vi "CAEN_daisy_isolated.vi"() -> ()   [LabVIEW 2018]
uses:
  <instrlib>/CAEN PSM/CAEN PSM.lvlib
panel:
  in  "Current Limit (0.00 uA)":sgl[](array[numeric]) format="%.2g"
  in  "Voltage Max (0.0 V)":u16[](array[numeric]) max=9999
  in  "Voltage Level (0.0 V)":dbl[](array[numeric]) format="%.1g"
  in  "Apply settings":bool
  out "IMon values (uA)":dbl[](array[numeric])
  out "VMon values (V)":dbl[](array[numeric])
  in  "stop":bool
  in  "VISA resource name":refnum<visa-resource-name>
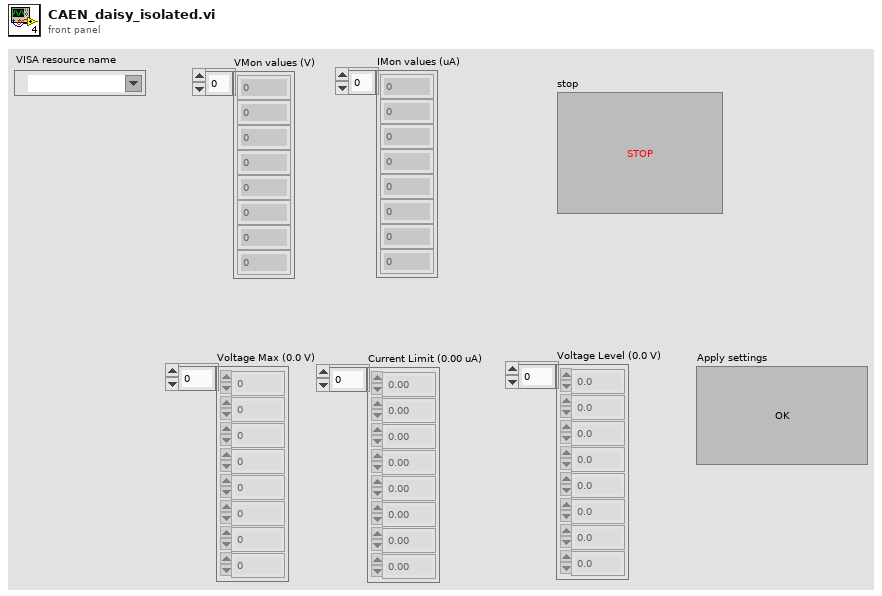
[diagram p1: front panel]
types:
  T1 = typedef "CAEN PSM.lvlib/BoardHandle.ctl" = cluster{"VISA resource name":refnum<visa-resource-name>, "Board address":u8, "NChannels":u8}
  T2 = cluster{"VISA resource name":refnum<visa-resource-name>, "Board address":u8, "NChannels":u8}
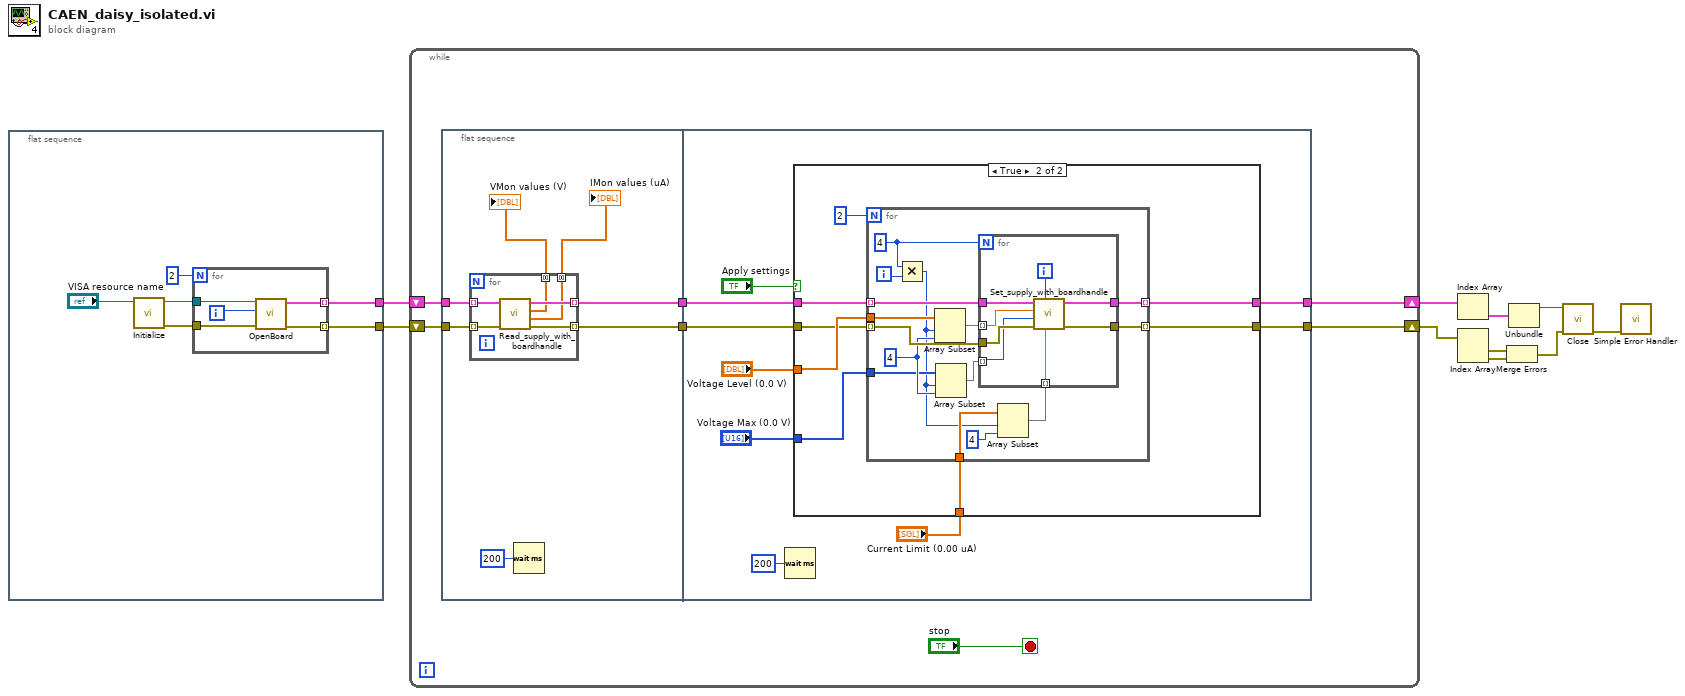
[diagram p0: block diagram]
diagram:
  n1 = flat-sequence {
    tunnel: [w12] -> w10
    tunnel: [w11] -> w9
    frame #0 {
      n2 = call <instrlib>:"Initialize.vi"("VISA resource name"="VISA resource name") -> ("error out"=w14:errorcluster, "VISA resource name out"=w15:refnum<visa-resource-name>)  [unwired: 9 in]
      n3 = for {
        N: 2 -> [_]
        tunnel: w15 -> [w21]
        tunnel: w14 -> [w19]
        tunnel: [w18] -> w11 mode=indexing
        tunnel: [w17] -> w12 mode=indexing
        i -> [w20]
        n4 = call <instrlib>:"OpenBoard.vi"("error in (no error)"=w19, "Board Address"=w20, "VISA resource name"=w21) -> ("error out"=w18:errorcluster, "BoardHandle"=w17:T1)  [unwired: 7 in]
      }
    }
  }
  n5 = while {
    shift-right: [w23] -> w8
    shift-left: w10 -> [w28]
    shift-right: [w22] -> w5
    shift-left: w9 -> [w27]
    stop <- "stop" stop-if-true
    n6 = flat-sequence {
      tunnel: w28 -> [w35]
      tunnel: w27 -> [w34]
      tunnel: [w33] -> w26
      tunnel: [w32] -> w25
      tunnel: w26 -> [w49]
      tunnel: w25 -> [w48]
      tunnel: [w47] -> w23
      tunnel: [w46] -> w22
      frame #0 {
        n7 = for {
          tunnel: w35 -> [w41] mode=indexing
          tunnel: w34 -> [w40] mode=indexing
          tunnel: [w39] -> w33 mode=indexing
          tunnel: [w38] -> w32 mode=indexing
          tunnel: [w37] -> w31 mode=concatenating
          tunnel: [w36] -> w30 mode=concatenating
          n8 = call "Read_supply_with_boardhandle.vi"("error in (no error)"=w40, "BoardHandle"=w41) -> ("error out"=w38:errorcluster, "IMon values (uA)"=w36:dbl[], "VMon values (V)"=w37:dbl[], "BoardHandle out"=w39:T2)  [unwired: 6 in]
        }
        "VMon values (V)" <- w31
        "IMon values (uA)" <- w30
        n9 = Wait (ms)(milliseconds to wait=u32 200) -> ()  [unwired: 1 out]
      }
      frame #1 {
        n10 = Wait (ms)(milliseconds to wait=u32 200) -> ()  [unwired: 1 out]
        n11 = case shown="True" "Apply settings" {
          tunnel: w49 -> [w52 w59]
          tunnel: w48 -> [w51 w56]
          tunnel: [w52 w58] -> w47
          tunnel: [w51 w55] -> w46
          tunnel: "Voltage Level (0.0 V)" -> [_ w60]
          tunnel: "Voltage Max (0.0 V)" -> [_ w54]
          tunnel: "Current Limit (0.00 uA)" -> [_ w53]
          frame False {
          }
          frame True {
            n12 = for {
              N: 2 -> [_]
              tunnel: w60 -> [w73]
              tunnel: w59 -> [w75] mode=indexing
              tunnel: [w74] -> w58 mode=indexing
              tunnel: w56 -> [w69] mode=indexing
              tunnel: [w68] -> w55 mode=indexing
              tunnel: w54 -> [w66]
              tunnel: w53 -> [w64]
              i -> [w71]
              w67 = 4 ("length")
              w72 = 4
              n13 = Multiply(x=w72, y=w71) -> (x*y=w63:i32)
              n14 = Array Subset(array=w73, index=w63, length=w67) -> (w70:dbl[])
              n15 = Array Subset(array=w66, index=w63, length=w67) -> (w65:u16[])
              n16 = Array Subset(array=w64, index=w63, length=4) -> (w61:sgl[])
              n17 = for {
                N: w72 -> [_]
                tunnel: w75 -> [w82]
                tunnel: [w81] -> w74
                tunnel: w70 -> [w80] mode=indexing
                tunnel: w69 -> [w79]
                tunnel: [w78] -> w68
                tunnel: w65 -> [w77] mode=indexing
                tunnel: w61 -> [w76] mode=indexing
                i -> [w83]
                n18 = call "Set_supply_with_boardhandle.vi"("Current Limit (0.00 uA)"=w76, "Channel (0)"=w83, "error in (no error)"=w79, "Voltage Max (0.0 V)"=w77, "Voltage Level (0.0 V)"=w80, "BoardHandle"=w82) -> ("error out"=w78:errorcluster, "BoardHandle out"=w81:T2)  [unwired: 4 in]
              }
            }
          }
        }
      }
    }
  }
  n19 = Index Array(array=w8) -> (element=w7:T1)  [unwired: 1 in]
  n20 = Index Array(array=w5) -> (element #1=w4:errorcluster, element #2=w3:errorcluster)  [unwired: 2 in]
  n21 = Merge Errors(w4, w3) -> (w2:errorcluster)
  n22 = Unbundle(w7) -> ("VISA resource name"=w6:refnum<visa-resource-name>)  [unwired: 2 out]
  n23 = call <instrlib>:"Close.vi"("error in (no error)"=w2, "VISA resource name"=w6) -> ("error out"=w1:errorcluster)  [unwired: 9 in]
  n24 = call <vilib>:"Simple Error Handler.vi"("error in (no error)"=w1) -> ()  [unwired: 4 in, 5 out]
